vi "Display Oval.vi"(4 "Brightness":u8=50 min=1 step=1, 6 "Factor":dbl=1.0, 8 "error in (no error)":errorcluster, 9 "Cluster":T1, 11 "Refnum in":refnum<k20>) -> (0 "error out":errorcluster, 3 "Refnum out":refnum<k20>, 5 "LED Matrix":picture)   [LabVIEW 2013]
uses:
  Cluser.ctl
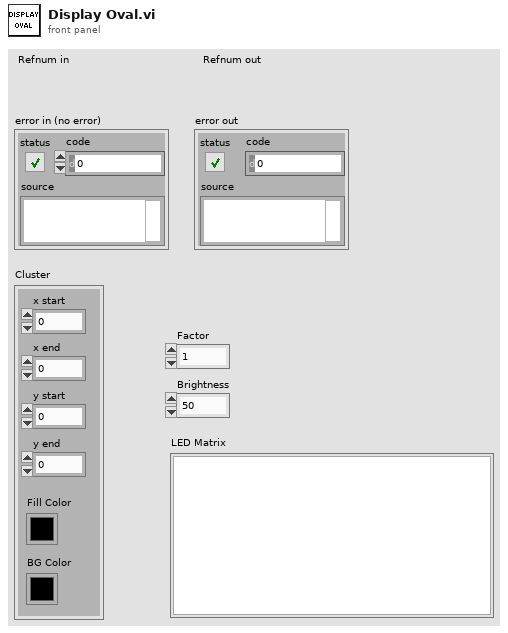
[diagram p1: front panel]
types:
  T1 = typedef "Cluser.ctl" = cluster{"x start":u16, "x end":u16, "y start":u16, "y end":u16, "Fill Color":u32, "BG Color":u32}
  T2 = cluster{"Left":i32, "Top":i32, "Right":i32, "Bottom":i32}
  T3 = typedef "Image Type" = u32
  T4 = typedef "IMAQ Image.ctl" = refnum<image>
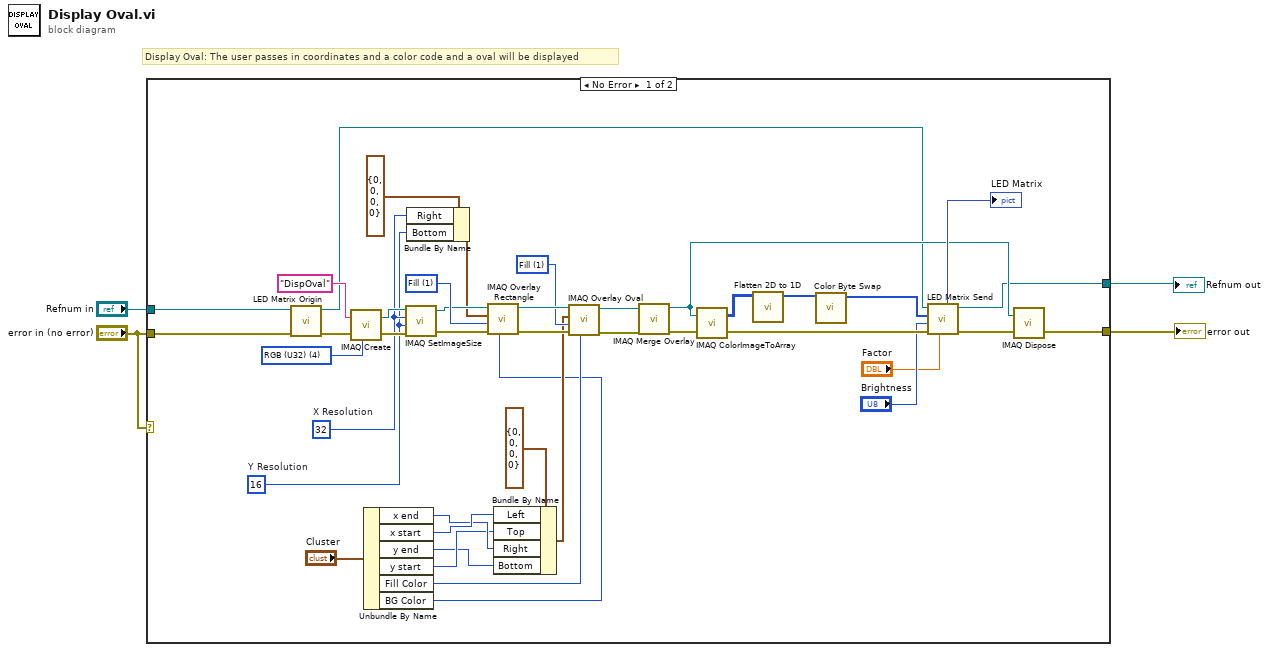
[diagram p0: block diagram]
diagram:
  # "Display Oval: The user passes in coordinates and a color code and a oval will be displayed"
  n1 = case shown="No Error" "error in (no error)" {
    tunnel: "error in (no error)" -> [w20 w46]
    tunnel: "Refnum in" -> [w19 w47]
    tunnel: [w27 w47] -> w1
    tunnel: [w26 w46] -> w3
    frame No Error {
      w14 = u32 1 items=["Frame", "Fill"] ("Drawing Mode (Frame)")
      w41 = u32 1 items=["Frame", "Fill", "Highlight"] ("Drawing Mode (Frame)")
      w21 = 16  # Y Resolution
      w22 = 32  # X Resolution
      w32 = T3 4 items=["Grayscale (U8)", "Grayscale (I16)", "Grayscale (SGL)", "Complex (CSG)", "RGB (U32)", "HSL (U32)", "RGB (U64)", "Grayscale (U16)"] ("Image Type")
      n2 = call "LED Matrix Origin.vi"("error in (no error)"=w20, "Refnum in"=w19) -> ("error out"=w31:errorcluster, "Refnum out"=w28:refnum<k20>)  [unwired: 8 in]
      n3 = call "IMAQ Create"("Image Name"="DispOval", "Image Type"=w32, "error in (no error)"=w31) -> ("New Image"=w35:T4, "error out"=w36:errorcluster)  [unwired: 2 in]
      n4 = Unbundle By Name("Cluster") -> ("x end"=w8:u16, "x start"=w9:u16, "y end"=w6:u16, "y start"=w7:u16, "Fill Color"=w12:u32, "BG Color"=w5:u32)
      n5 = call "IMAQ SetImageSize"("error in (no error)"=w36, "Y Resolution"=w21, "X Resolution"=w22, "Image"=w35) -> ("error out"=w40:errorcluster, "Image Out"=w39:T4)  [unwired: 1 in]
      n6 = Bundle By Name(cluster=T2 {"Left"=0, "Top"=0, "Right"=0, "Bottom"=0} ("Rectangle"), "Right"=w22, "Bottom"=w21) -> (w24:T2)
      n7 = call "IMAQ Overlay Rectangle"("Color"=w5, "error in (no error)"=w40, "Drawing Mode (Frame)"=w41, "Rectangle"=w24, "Image"=w39) -> ("error out"=w16:errorcluster, "Image Out"=w18:T4)  [unwired: 5 in]
      n8 = Bundle By Name(cluster=T2 {"Left"=0, "Top"=0, "Right"=0, "Bottom"=0} ("Bounding Rectangle"), "Left"=w9, "Top"=w7, "Right"=w8, "Bottom"=w6) -> (w10:T2)
      n9 = call "IMAQ Overlay Oval"("Color"=w12, "error in (no error)"=w16, "Drawing Mode (Frame)"=w14, "Bounding Rectangle"=w10, "Image"=w18) -> ("error out"=w15:errorcluster, "Image Out"=w17:T4)  [unwired: 5 in]
      n10 = call "IMAQ Merge Overlay"("error in (no error)"=w15, "Image Src"=w17) -> ("error out"=w42:errorcluster, "Image Dst Out"=w43:T4)  [unwired: 8 in]
      n11 = call "IMAQ ColorImageToArray"("Image"=w43, "error in (no error)"=w42) -> ("Image Pixels (U32)"=w34:u32[][], "error out"=w44:errorcluster)  [unwired: 2 in, 1 out]
      n12 = call "Flatten 2D to 1D.vi"("Image Pixels (U32) in"=w34) -> ("Image Pixels (U32) out"=w37:u32[])  [unwired: 10 in]
      n13 = call "Color Byte Swap.vi"("Image Pixels (U32) in"=w37) -> ("Images Pixels Out"=w38:u32[])  [unwired: 10 in]
      n14 = call "LED Matrix Send.vi"("Gamma"="Factor", "error in (no error)"=w44, "Brightness"="Brightness", "Data"=w38, "Refnum in"=w28) -> ("error out"=w30:errorcluster, "Refnum out"=w27:refnum<k20>, "LED Matrix"=→"LED Matrix":picture)  [unwired: 3 in]
      n15 = call "IMAQ Dispose"("Image"=w43, "error in (no error)"=w30) -> ("error out"=w26:errorcluster)  [unwired: 4 in]
    }
    frame Error {
    }
  }
  "error out" <- w3
  "Refnum out" <- w1
